vi "Tool Object.vi"(8 "error in (no error)":errorcluster, 11 "Tool Rectangle in":refnum<class "Tool Rectangle.lvclass">) -> (0 "error out":errorcluster, 3 "Tool Rectangle out":refnum<class "Tool Rectangle.lvclass">)   [LabVIEW 2019, in "Tool Rectangle.lvclass"]
uses:
  Tool Rectangle.lvclass
  Settings/ObjectSettings/ObjectSettings.lvclass/ObjectSettings.ctl
  Settings/Rectangle Settings/Rectangle Settings.lvclass
  C:/Users/Albro/Documents/GitHub/AFM-Lithography/lvsrc/Classes/Settings/ObjectSettings/ObjectSettings.lvclass
  Settings/ObjectSettings/ObjectSettings.lvclass
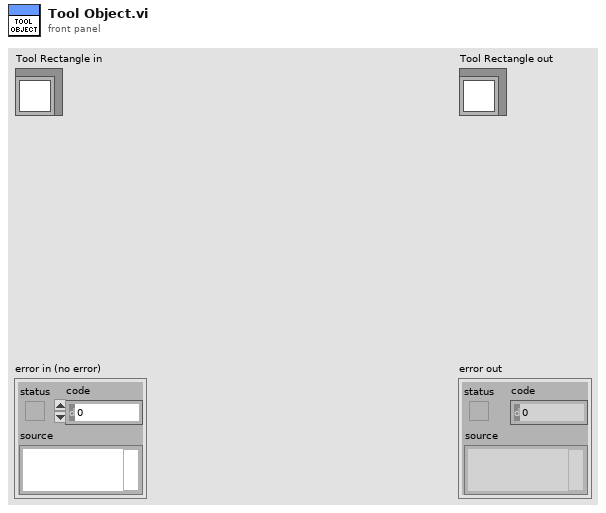
[diagram p1: front panel]
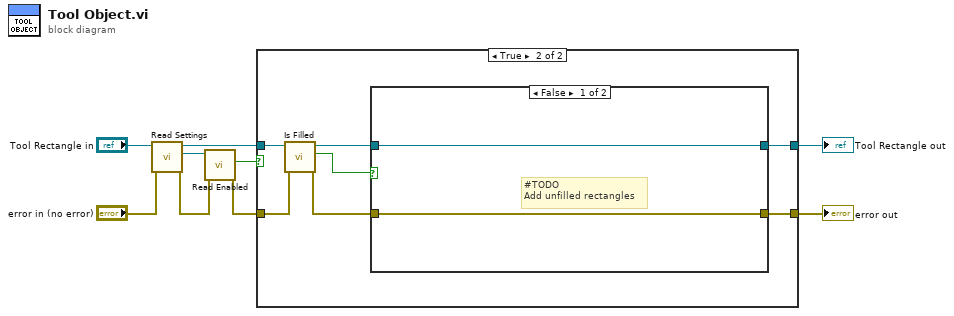
[diagram p0: block diagram]
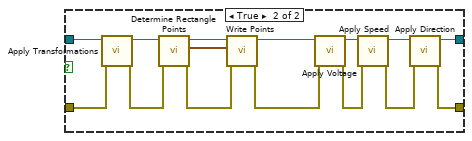
[diagram p3: hidden frame]
diagram:
  n1 = call-dynamic "Read Settings.vi"("error in (no error)"="error in (no error)", "Tool Rectangle in"="Tool Rectangle in") -> ("error out"=w4:errorcluster, "Rectangle Settings.lvclass"=w5:refnum<class "Rectangle Settings.lvclass">, "Tool Rectangle out"=w6:refnum<class "Tool Rectangle.lvclass">)  [unwired: 7 in]
  n2 = call "Read Enabled.vi"("error in (no error)"=w4, "ObjectSettings in"=w5) -> ("error out"=w8:errorcluster, "Enabled"=w9:bool)  [unwired: 7 in, 1 out]
  n3 = case shown="True" w9 {
    tunnel: w6 -> [w11 w18]
    tunnel: [w11 w16] -> w2
    tunnel: w8 -> [w10 w15]
    tunnel: [w10 w14] -> w1
    frame False {
    }
    frame True {
      n4 = call-dynamic "Is Filled.vi"("error in (no error)"=w15, "Tool Rectangle in"=w18) -> ("error out"=w13:errorcluster, "x != y?"=w12:bool, "Tool Rectangle out"=w17:refnum<class "Tool Rectangle.lvclass">)  [unwired: 7 in]
      n5 = case shown="False" w12 {
        tunnel: w17 -> [w20 w35]
        tunnel: [w20 w26] -> w16
        tunnel: [w19 w21] -> w14
        tunnel: w13 -> [w19 w34]
        frame False {
          # "#TODO\nAdd unfilled rectangles"
        }
        frame True {
          n6 = call-dynamic "Apply Transformations.vi"("error in (no error)"=w34, "Tool Rectangle in"=w35) -> ("error out"=w32:errorcluster, "Tool Rectangle out"=w33:refnum<class "Tool Rectangle.lvclass">)  [unwired: 8 in]
          n7 = call-dynamic "Determine Rectangle Points.vi"("error in (no error)"=w32, "Tool Rectangle in"=w33) -> ("error out"=w29:errorcluster, "interleaved array"=w30:cluster{"X":dbl, "Y":dbl}[], "Tool Rectangle out"=w31:refnum<class "Tool Rectangle.lvclass">)  [unwired: 7 in]
          n8 = call-dynamic "Write Points.vi"("error in (no error)"=w29, "Points"=w30, "Tool Object in"=w31) -> ("error out"=w24:errorcluster, "Tool Object out"=w28:refnum<class "Tool Rectangle.lvclass">)  [unwired: 7 in]
          n9 = call-dynamic "Apply Voltage.vi"("error in (no error)"=w24, "Tool Rectangle in"=w28) -> ("error out"=w23:errorcluster, "Tool Rectangle out"=w27:refnum<class "Tool Rectangle.lvclass">)  [unwired: 8 in]
          n10 = call-dynamic "Apply Speed.vi"("error in (no error)"=w23, "Tool Rectangle in"=w27) -> ("error out"=w22:errorcluster, "Tool Rectangle out"=w25:refnum<class "Tool Rectangle.lvclass">)  [unwired: 8 in]
          n11 = call-dynamic "Apply Direction.vi"("error in (no error)"=w22, "Tool Rectangle in"=w25) -> ("error out"=w21:errorcluster, "Tool Rectangle out"=w26:refnum<class "Tool Rectangle.lvclass">)  [unwired: 8 in]
        }
      }
    }
  }
  "error out" <- w1
  "Tool Rectangle out" <- w2
